vi "运维调试_氨氮.vi"() -> ()   [LabVIEW 2016, in "氨氮.lvlib"]
uses:
  <vilib>/Platform/TimedLoop/XDataNode/timing_clust.ctl
  <vilib>/Platform/TimedLoop/XDataNode/nitl_modes.ctl
  <vilib>/Platform/TimedLoop/XDataNode/wakeup.ctl
  <vilib>/Utility/miscctls.llb/LVPointTypeDef.ctl
  <vilib>/Platform/TimedLoop/XDataNode/XDataNode.xnode
  <vilib>/Platform/TimedLoop/XDataNode/XDNodeRunTimeDep.lvlib
panel:
  in  "设置":bool
  in  "返回 2":bool
  out "固件版本号":string
  in  "数组":string[](array[string])
  in  "备用系数写入":bool
  in  "备用系数读取":bool
  in  "备用系数":T1
  in  "量程切换阈值写入":bool
  in  "量程切换阈值读取":bool
  in  "量程切换阈值":cluster{"阈值":dbl, "标液浓度":dbl}
  in  "参数下拉列表":enum16{"氨氮", "总磷"}(ring)
  in  "量程下拉列表":enum16{"低量程", "高量程"}(ring)
  in  "测量模式下拉列表":enum16{"水样测量", "空白核查", "标样核查", "盲样测试", "加标回收"}(ring)
  in  "公式":cluster{"X^2":dbl, "X":dbl, "b":dbl}
  in  "写公式":bool
  in  "读公式":bool
  in  "精度":dbl=4.0
  in  "样品5 F0":dbl
  in  "样品5 F1":dbl
  in  "样品4 F1":dbl
  in  "样品4 F0":dbl
  in  "样品3 F0":dbl
  in  "样品3 F1":dbl
  in  "样品2 F0":dbl
  in  "样品2 F1":dbl
  in  "样品1 F1":dbl
  in  "样品1 F0":dbl
  in  "method":u16(ring) items=["最小二乘", "最小绝对残差", "Bisquare"]
  in  "模型":enum32{"线性", "多项式"}(ring)
  out "r^2":dbl format="%.7g"
  out "拟合公式":string
  in  "样品2启用":bool
  in  "样品5启用":bool
  in  "样品4启用":bool
  in  "样品3启用":bool
  in  "样品1启用":bool
  in  "标液浓度5":dbl
  out "测量吸光度5":dbl
  in  "标液浓度4":dbl
  out "测量吸光度4":dbl
  in  "标液浓度3":dbl
  out "测量吸光度3":dbl
  in  "标液浓度2":dbl
  out "测量吸光度2":dbl
  out "测量吸光度1":dbl
  in  "标液浓度1":dbl
  out "XY图":cluster{"X Values":dbl[], "Y Values":dbl[]}[](graph)
  in  "返回":bool
  in  "调试":bool
  out "序列号":string="序列号"
  out "氨氮测量数据":T2(xcontrol)
  out "集成报警信息":string
  out "设置值":dbl
  out "定时启动":bool
  out "总磷总氮运行状态":T3(xcontrol)
  in  "停止":bool
  in  "手动启动":bool
  in  "单步测试":bool
  in  "总磷氨氮调试":u16[](xcontrol)
  out "F3":sgl format="%#.6f"
  out "F2":sgl format="%#.6f"
  out "F1":sgl format="%#.6f"
  out "F0":sgl format="%#.6f"
  out "多列列表框":i32(listbox)
  # "COM1"
  # "参数设置"
  # "标液浓度"
  # "F0"
  # "F1"
  # "吸光值显示"
  # "辅\n助\n计\n算\n区"
  # "样品一"
  # "样品二"
  # "样品三"
  # "样品四"
  # "样品五"
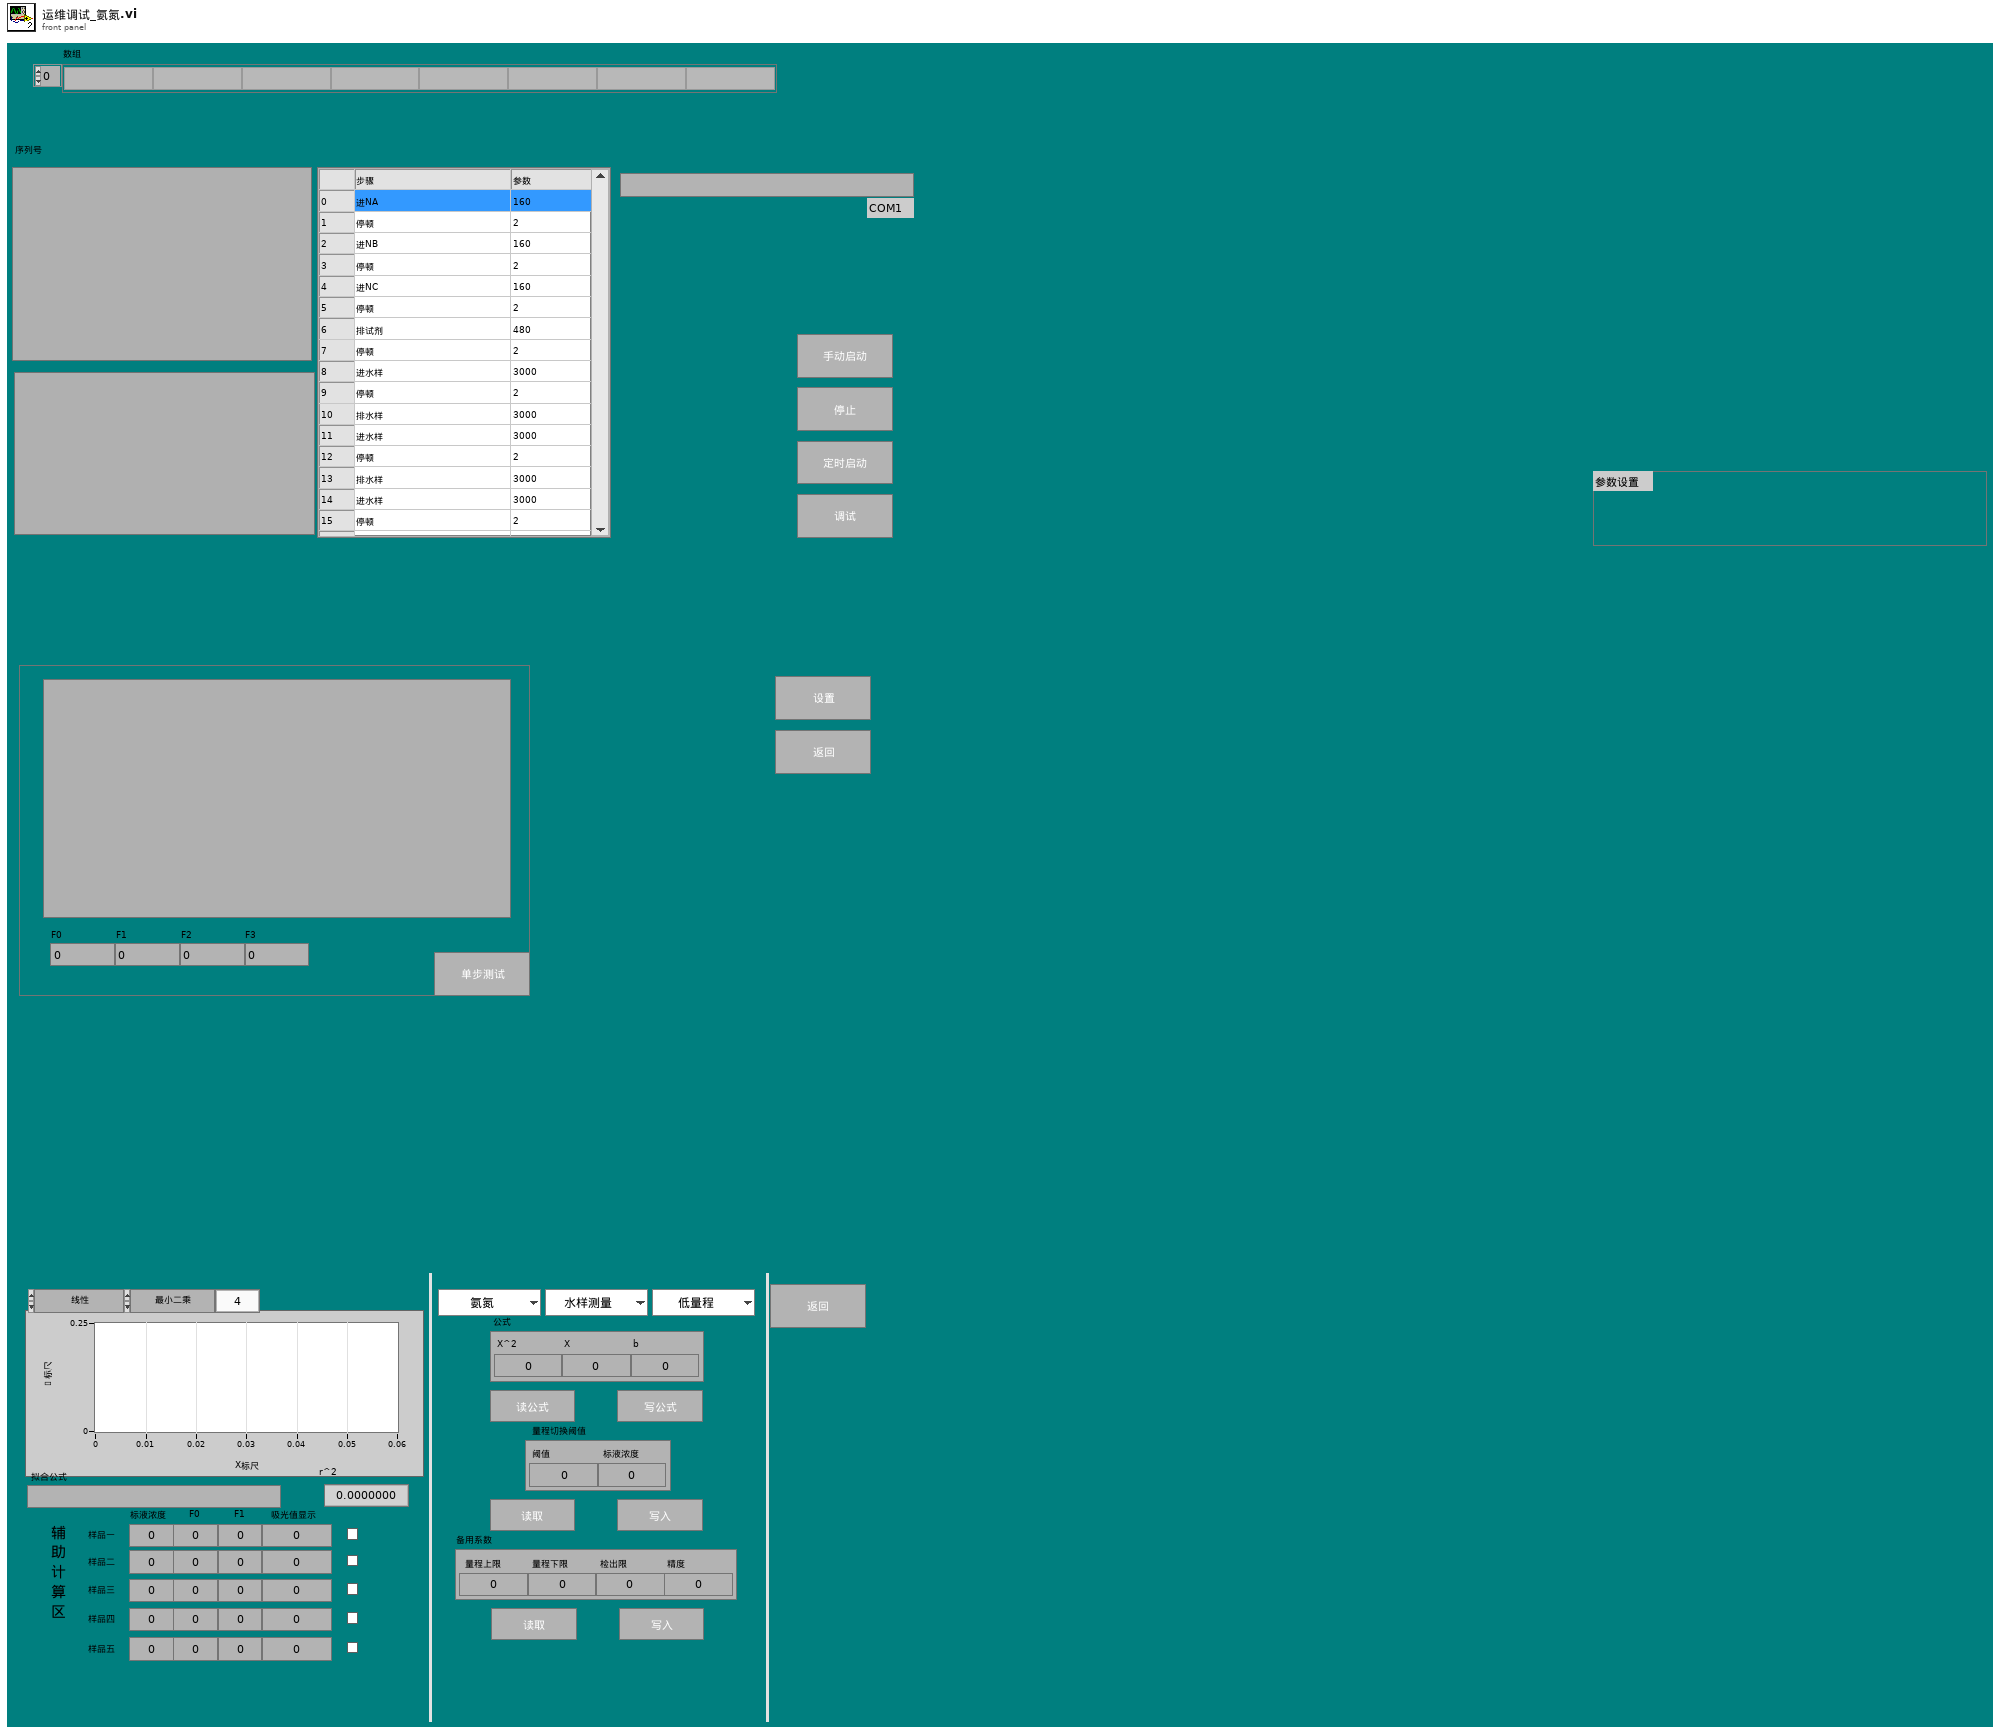
[diagram p1: front panel]
types:
  T1 = cluster{"量程上限":dbl, "量程下限":dbl, "检出限":dbl, "精度":dbl}
  T2 = cluster{"flowid":u16, "测量精度":u16, "测量数据区":cluster{"因子编码":u32, "单位":u16, "标样参考值":sgl, "水样数据时间":timestamp, "水样实测值":sgl, "水样数据标识":string, "标样数据时间":timestamp, "标样实测值":sgl, "标样数据标识":string, "空白数据时间":timestamp, "空白实测值":sgl, "空白数据标识":string, "零点核查数据时间":timestamp, "零点核查实测值":sgl, "零点核查数据标识":string, "跨度核查数据时间":timestamp, "跨度核查实测值":sgl, "跨度核查数据标识":string, "加标回收数据时间":timestamp, "加标回收实测值":sgl, "加标回收数据标识":string, "平行样数据时间":timestamp, "平行样实测值":sgl, "平行样数据标识":string}}
  T3 = cluster{"系统时间":timestamp, "工作状态":enum16{"空闲", "水样测试", "标样核查", "零点核查", "跨度核查", "空白测试", "平行样测试", "加标回收", "空白校准", "标样校准", "初始化（清洗）"}, "测量模式":enum16{"待机", "连续模式", "周期模式", "定点模式", "受控模式", "手动模式"}, "告警代码":enum16{"无告警", "缺试剂告警", "缺水样告警", "缺蒸馏水告警", "缺标液告警", "仪表漏液告警", "标定异常告警", "超量程告警", "加热异常", "低试剂预警", "超上限告警", "超下限告警", "仪表内部其他异常", "滴定异常告警", "电极异常告警", "量程切换告警", "参数设置告警", "PH电极电位异常", "电导率电极异常", "浊度光度异常", "溶解氧电极异常", "溶解氧光强异常", "温度异常告警", "PH异常告警", "溶解氧异常告警", "电导率异常告警", "浊度异常告警", "叶绿素异常告警", "藻密度异常告警", "蓝绿藻异常告警", "ORP异常告警", "氨氮异常告警", "清洁刷异常告警", "SD卡异常告警", "蓝牙异常告警", "Wifi异常告警", "流程异常告警"}, "故障代码":enum16{"无故障", "电机故障", "温度故障", "通讯故障", "滴定故障"}, "日志代码":u16, "软件版本":u16, "F0":sgl, "F1":sgl, "F2":sgl, "F3":sgl, "T":sgl, "H":sgl, "id":u16, "flowid":u16, "量程":u16}
  T4 = enum16{"待机", "启动氨氮", "氨氮测量中", "启动总磷", "总磷测量中", "延时"}
  T5 = typedef "LVPointTypeDef.ctl" = cluster{"Horizontal":i16, "Vertical":i16}
  T6 = cluster{"因子编码":u32, "单位":u16, "标样参考值":sgl, "水样数据时间":timestamp, "水样实测值":sgl, "水样数据标识":string, "标样数据时间":timestamp, "标样实测值":sgl, "标样数据标识":string, "空白数据时间":timestamp, "空白实测值":sgl, "空白数据标识":string, "零点核查数据时间":timestamp, "零点核查实测值":sgl, "零点核查数据标识":string, "跨度核查数据时间":timestamp, "跨度核查实测值":sgl, "跨度核查数据标识":string, "加标回收数据时间":timestamp, "加标回收实测值":sgl, "加标回收数据标识":string, "平行样数据时间":timestamp, "平行样实测值":sgl, "平行样数据标识":string}
  T7 = enum16{"空闲", "水样测试", "标样核查", "零点核查", "跨度核查", "空白测试", "平行样测试", "加标回收", "空白校准", "标样校准", "初始化（清洗）"}
  T8 = cluster{"启动模式":enum16{"标液测量", "水样测量", "零液测量", "盲样测量", "加标回收"}, "启动参数":u16, "量程":enum16{"低量程", "高量程"}}
  T9 = cluster{"时间标识":timestamp, "设备":string, "日志信息":string, "流程参数":string}
  T10 = cluster{"时间标识":timestamp, "设备":string, "日志信息":string}
  T11 = enum16{"无告警", "缺试剂告警", "缺水样告警", "缺蒸馏水告警", "缺标液告警", "仪表漏液告警", "标定异常告警", "超量程告警", "加热异常", "低试剂预警", "超上限告警", "超下限告警", "仪表内部其他异常", "滴定异常告警", "电极异常告警", "量程切换告警", "参数设置告警", "PH电极电位异常", "电导率电极异常", "浊度光度异常", "溶解氧电极异常", "溶解氧光强异常", "温度异常告警", "PH异常告警", "溶解氧异常告警", "电导率异常告警", "浊度异常告警", "叶绿素异常告警", "藻密度异常告警", "蓝绿藻异常告警", "ORP异常告警", "氨氮异常告警", "清洁刷异常告警", "SD卡异常告警", "蓝牙异常告警", "Wifi异常告警", "流程异常告警"}
  T12 = typedef "LVRowAndColumnUnsignedTypeDef.ctl" = cluster{"Row":u32, "Column":u32}
  T13 = typedef "XDNodeRunTimeDep.lvlib/timing_clust.ctl" = cluster{"Expected End [f-1]":u64, "Actual End [f-1]":u64, "Finished Late? [f-1]":bool, "Expected End [i-1]":u64, "Actual End [i-1]":u64, "Finished Late? [i-1]":bool, "Expected Start [i]":u64, "Actual Start [i]":u64, "Expected Start [f]":u64, "Actual Start [f]":u64, "Source Name":string, "Structure Name":string, "Period":i64, "Deadline":i64, "Offset":i64, "Start":i64, "Priority":i32, "Timeout":i32, "Mode":T14, "Wakeup Reason":T15, "Error":errorcluster, "Source Type":string, "Secondary Source Type":string, "Global End Time":u64, "Global Start Time":u64, "Frame Duration":u64, "Iteration Duration":u64, "Assigned CPU":i32, "I/O Scan Engine Mode":u32}
  T14 = typedef "XDNodeRunTimeDep.lvlib/nitl_modes.ctl" = enum32{"No Change", "Process missed periods, maintain original phase", "Discard missed periods, maintain original phase", "Process missed periods, ignore original phase", "Discard missed periods, ignore original phase"}
  T15 = typedef "XDNodeRunTimeDep.lvlib/wakeup.ctl" = enum32{"Normal", "Aborted", "Asynchronous wakeup", "Timing source error", "Timed loop error", "Timeout"}
  T16 = cluster{"站号":u16, "量程切换":enum32{"H", "L", "AUTO"}, "控制命令":enum16{"启动测量", "标样核查", "零点核查", "跨度核查", "空白测试", "平行样测试", "加标回收", "空白校准", "标样校准", "初始化（清洗）", "停止测试", "仪器重启", "校时", "模式设置", "测量间隔设置", "盲样测试"}, "模式设置":enum16{"待机", "连续模式", "周期模式", "定点模式", "受控模式", "手动模式"}, "测量间隔":u16}
  T17 = cluster{"站号":u16, "量程切换":enum32{"H", "L", "AUTO"}, "控制命令":enum16{"启动测量", "标样核查", "零点核查", "跨度核查", "空白测试", "平行样测试", "加标回收", "空白校准", "标样校准", "初始化（清洗）", "停止测试", "仪器重启", "校时", "模式设置", "测量间隔设置"}, "模式设置":enum16{"待机", "连续模式", "周期模式", "定点模式", "受控模式", "手动模式"}, "测量间隔":u16}
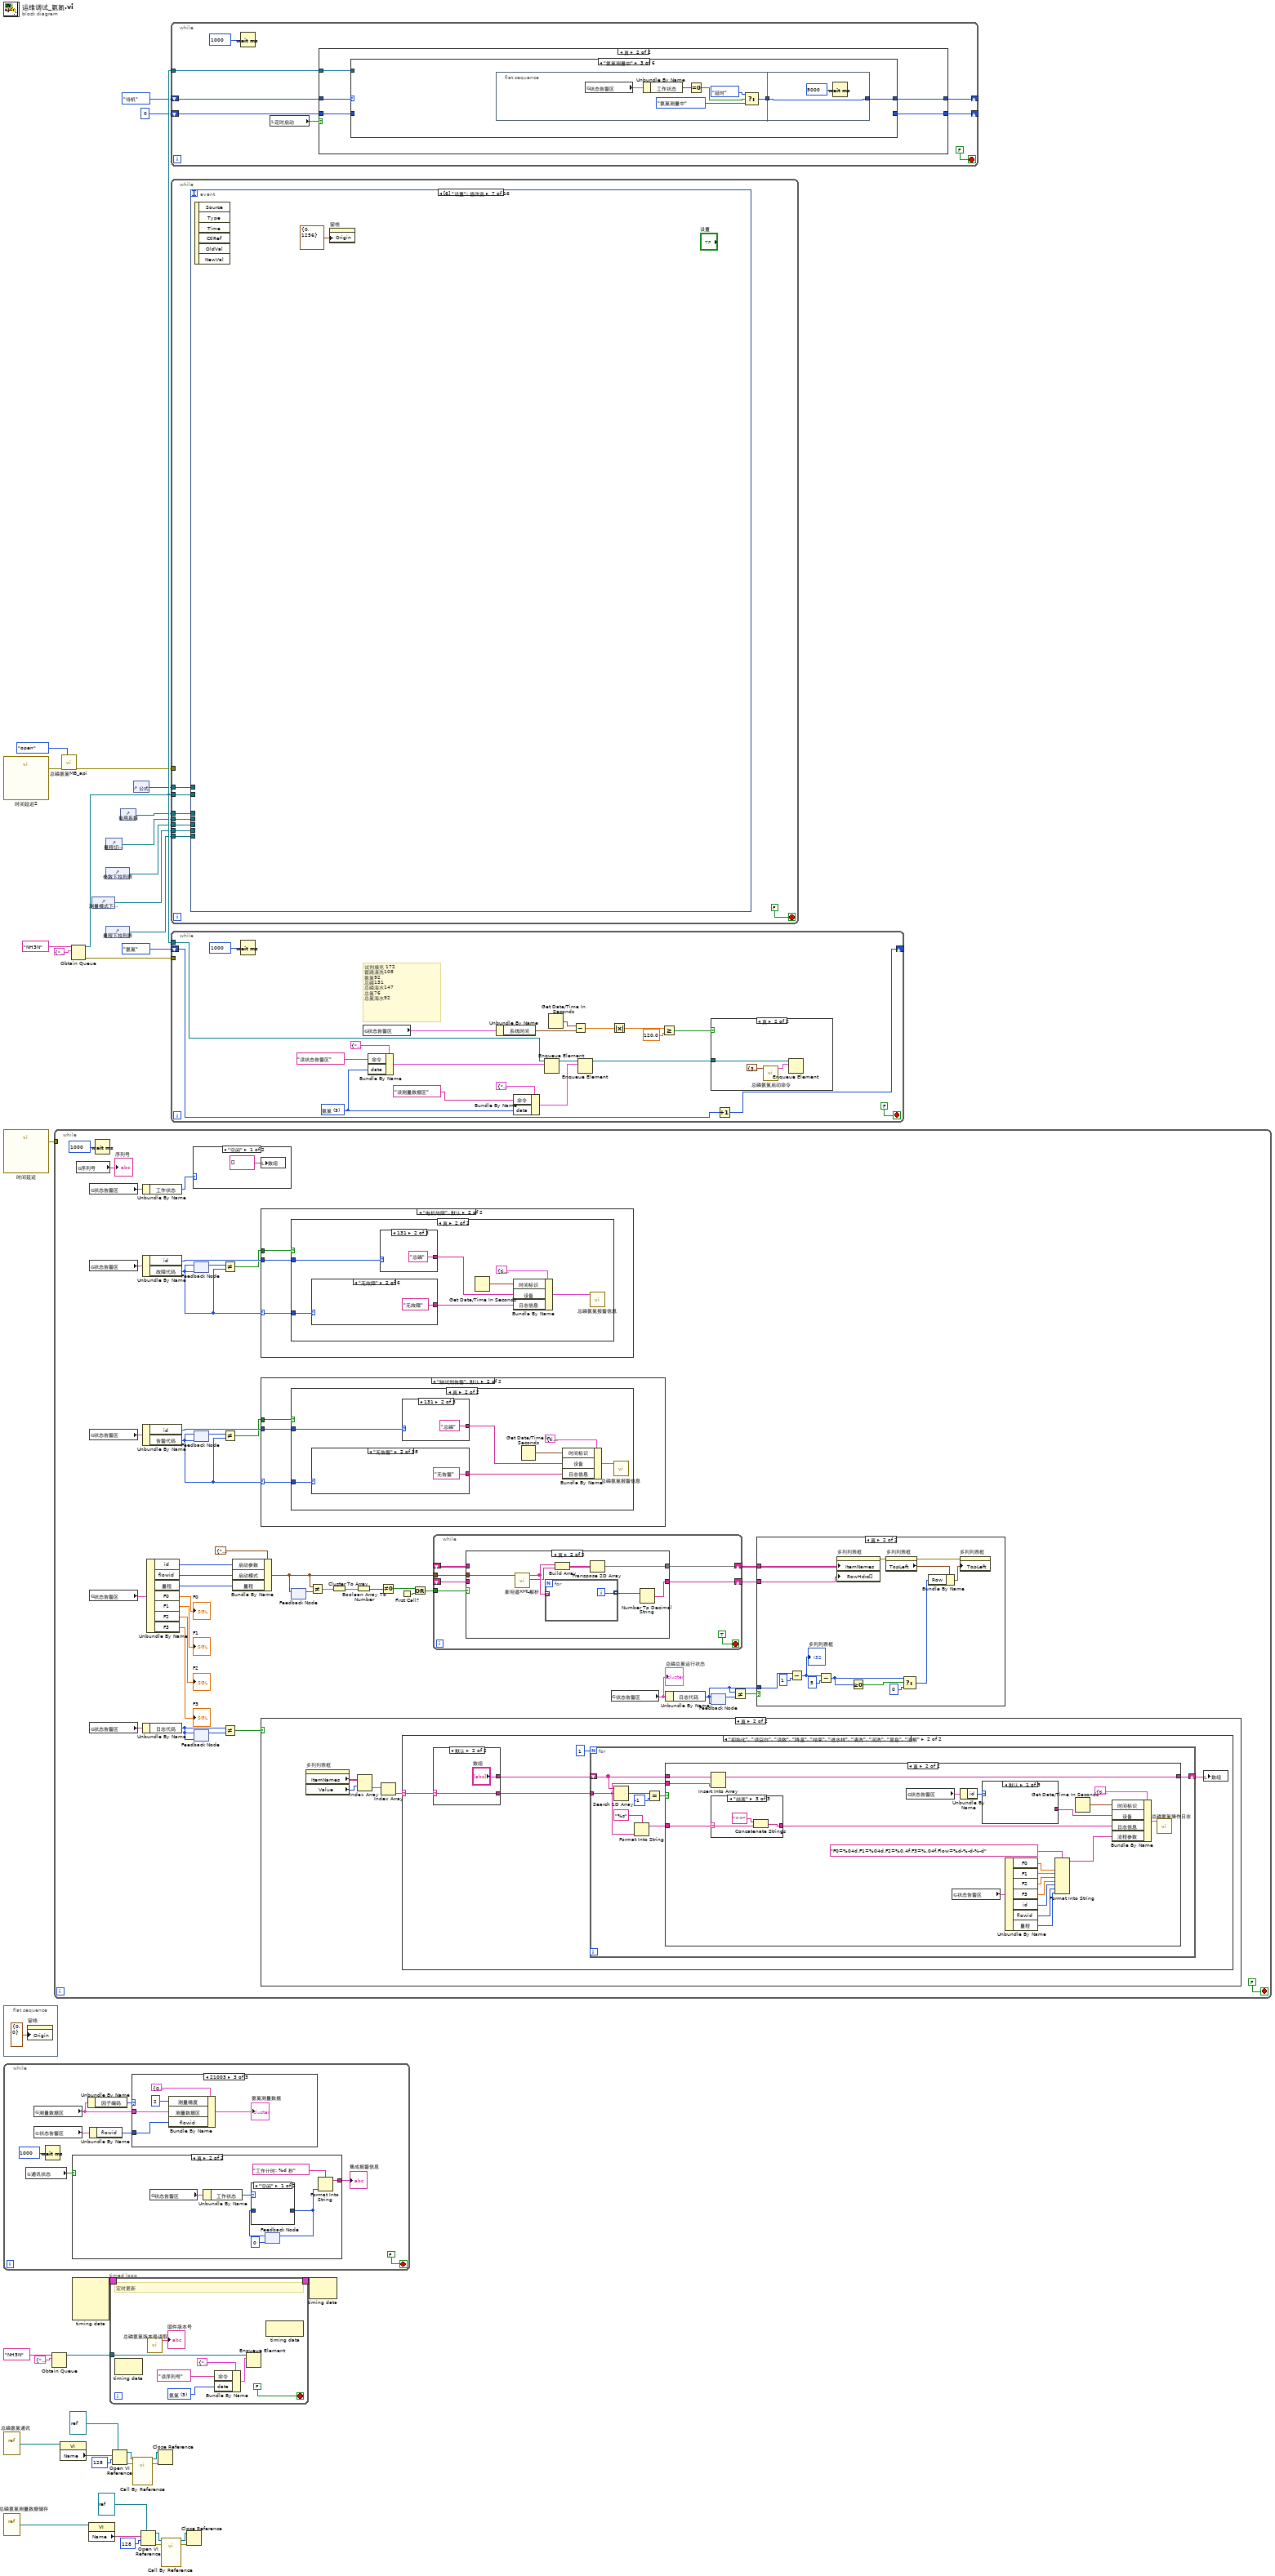
[diagram p0: block diagram]
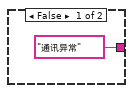
[diagram p2: hidden frame]
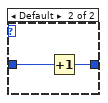
[diagram p3: hidden frame]
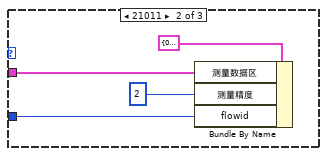
[diagram p5: hidden frame]
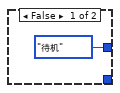
[diagram p6: hidden frame]
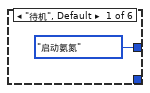
[diagram p7: hidden frame]
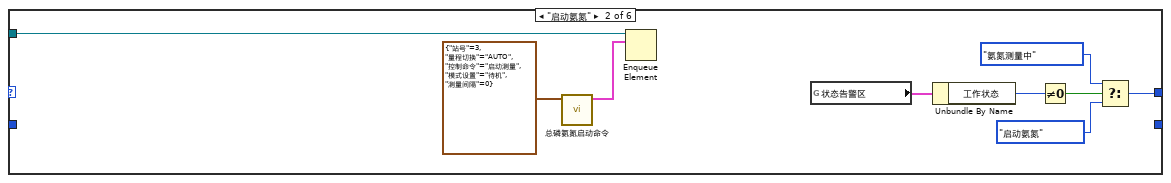
[diagram p8: hidden frame]
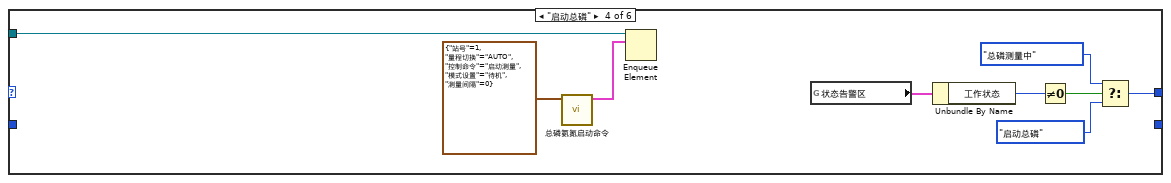
[diagram p9: hidden frame]
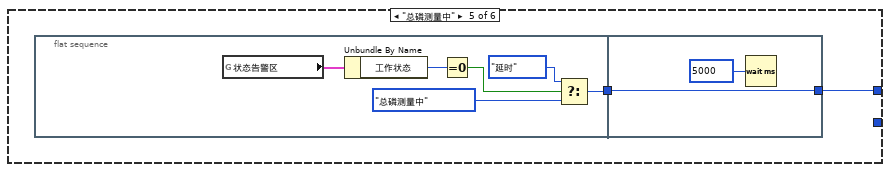
[diagram p10: hidden frame]
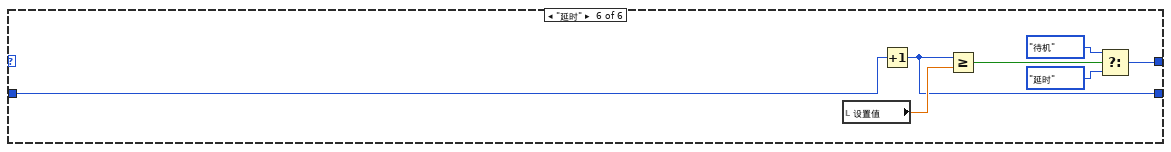
[diagram p11: hidden frame]
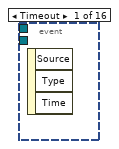
[diagram p12: hidden frame]
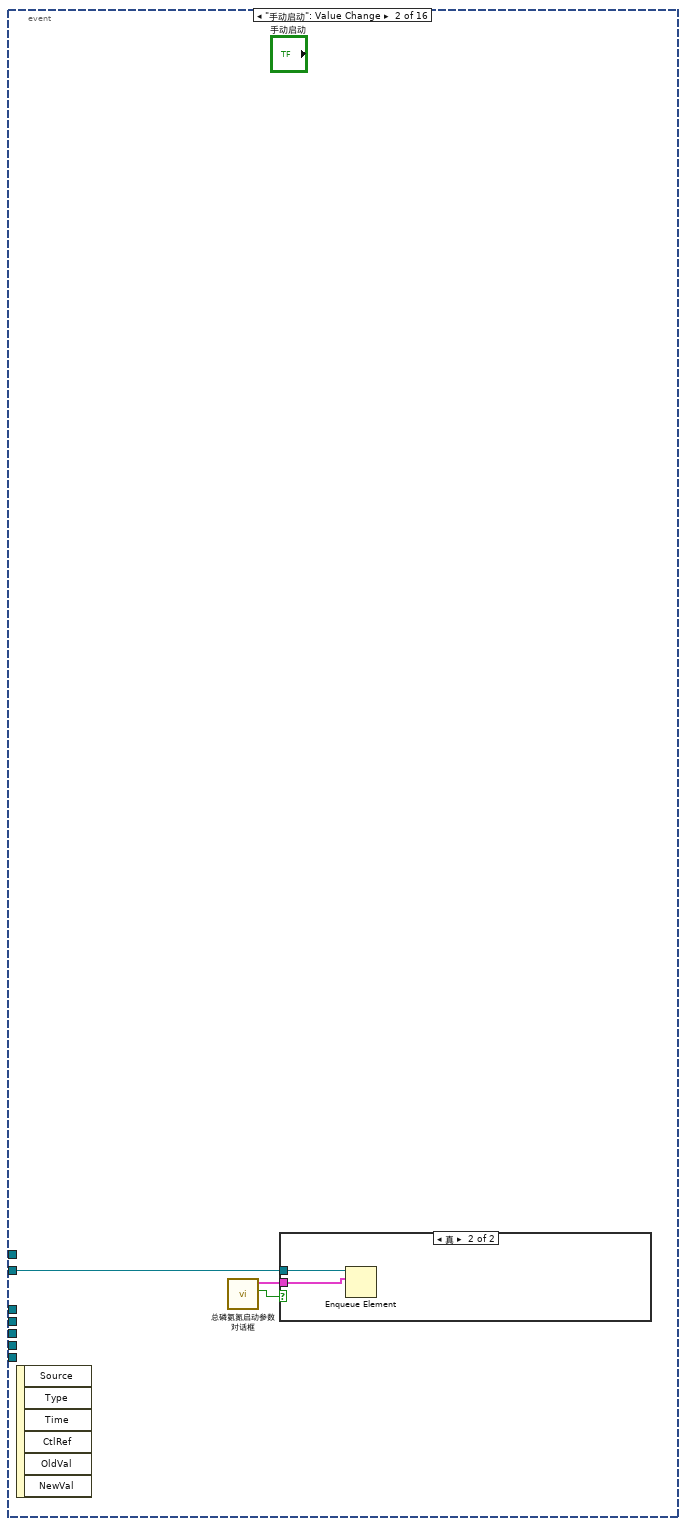
[diagram p13: hidden frame]
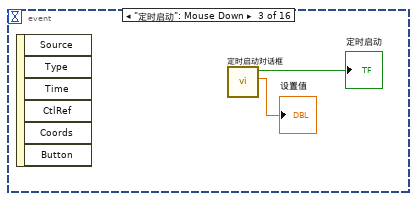
[diagram p15: hidden frame]
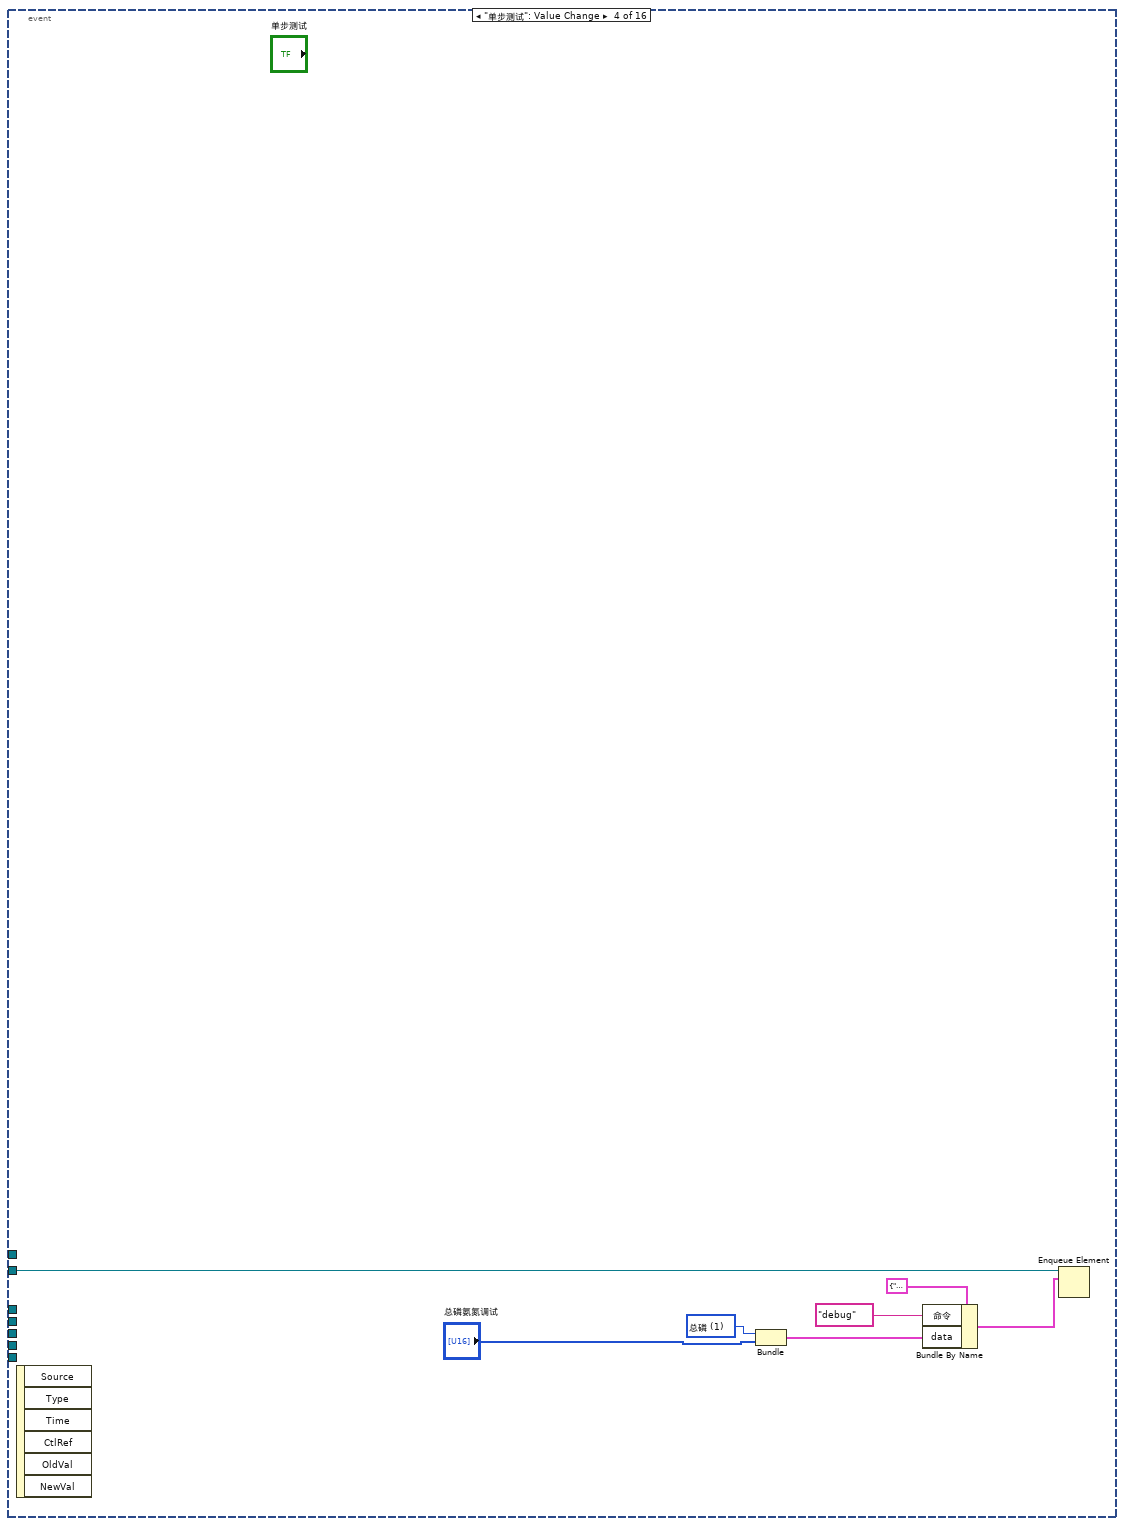
[diagram p16: hidden frame]
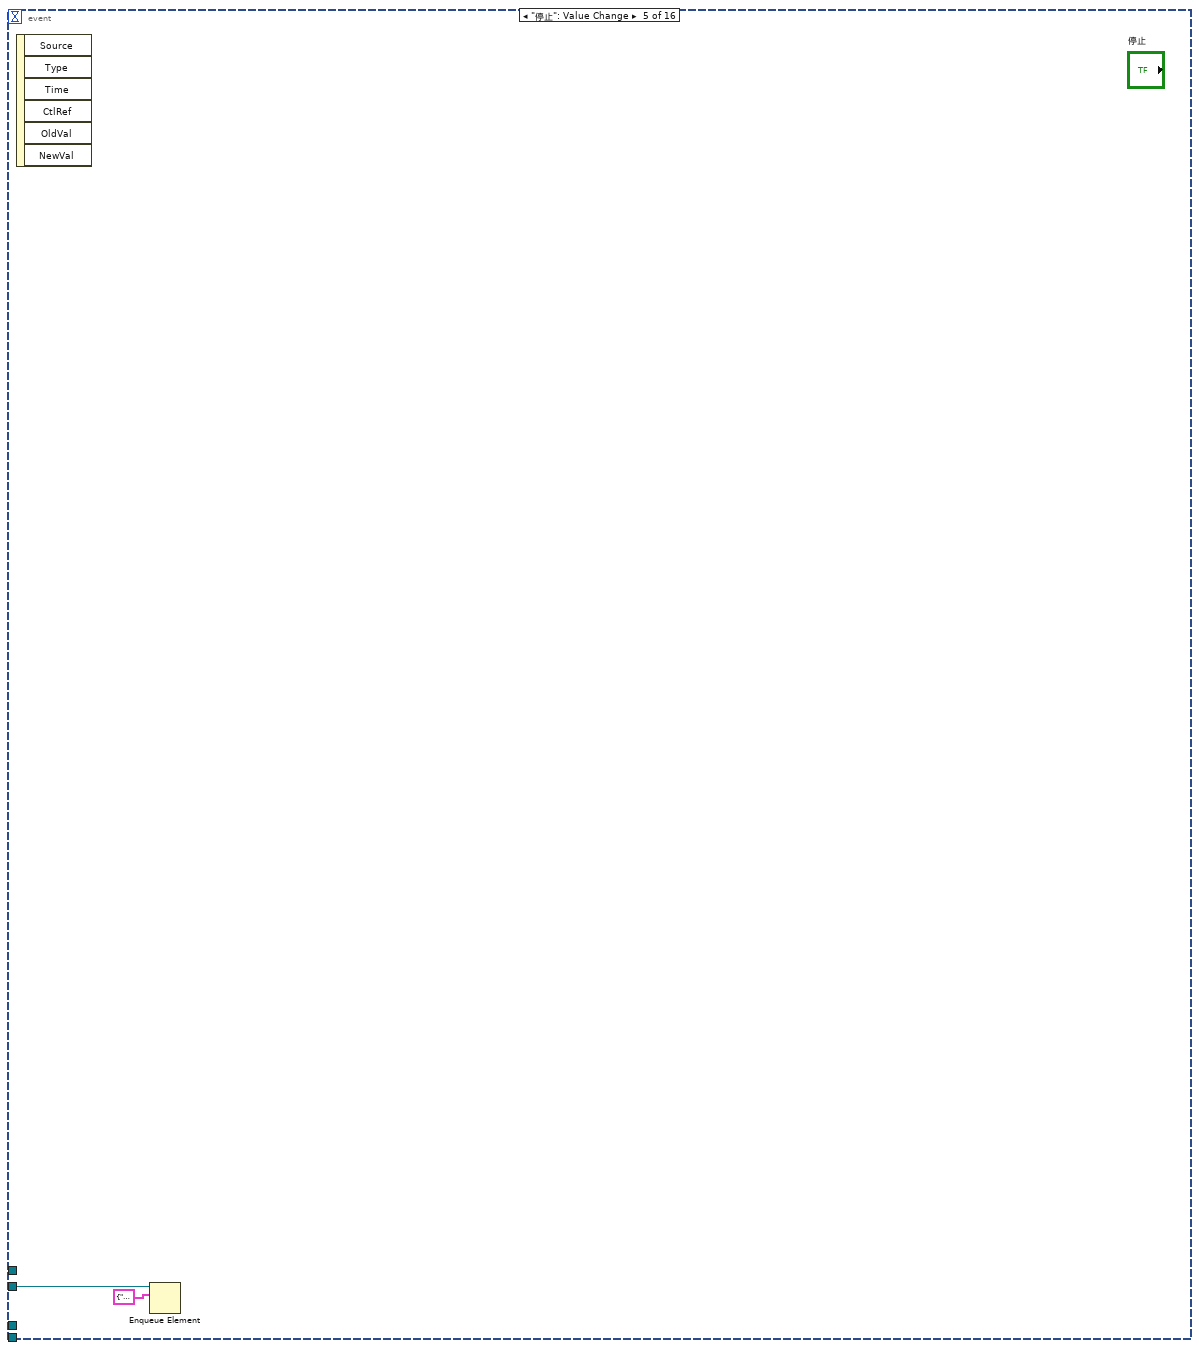
[diagram p17: hidden frame]
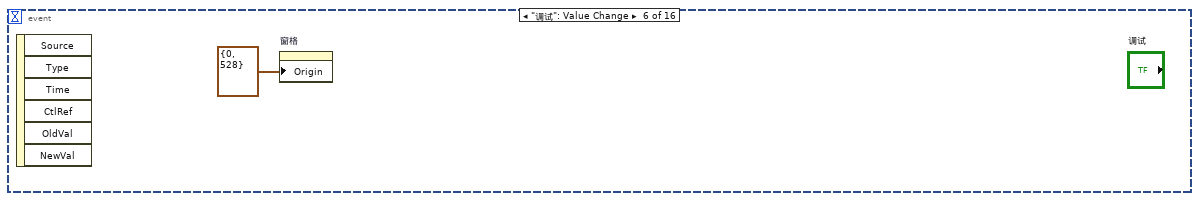
[diagram p18: hidden frame]
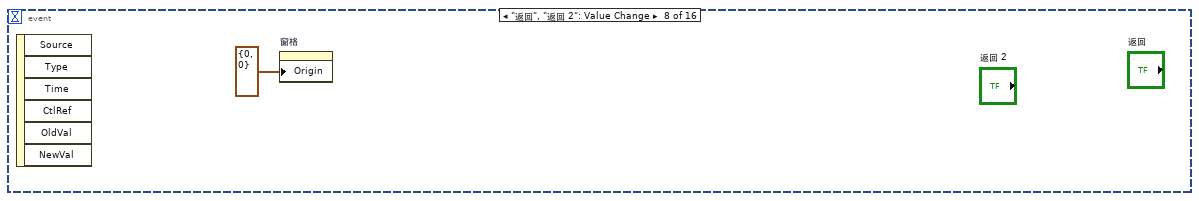
[diagram p19: hidden frame]
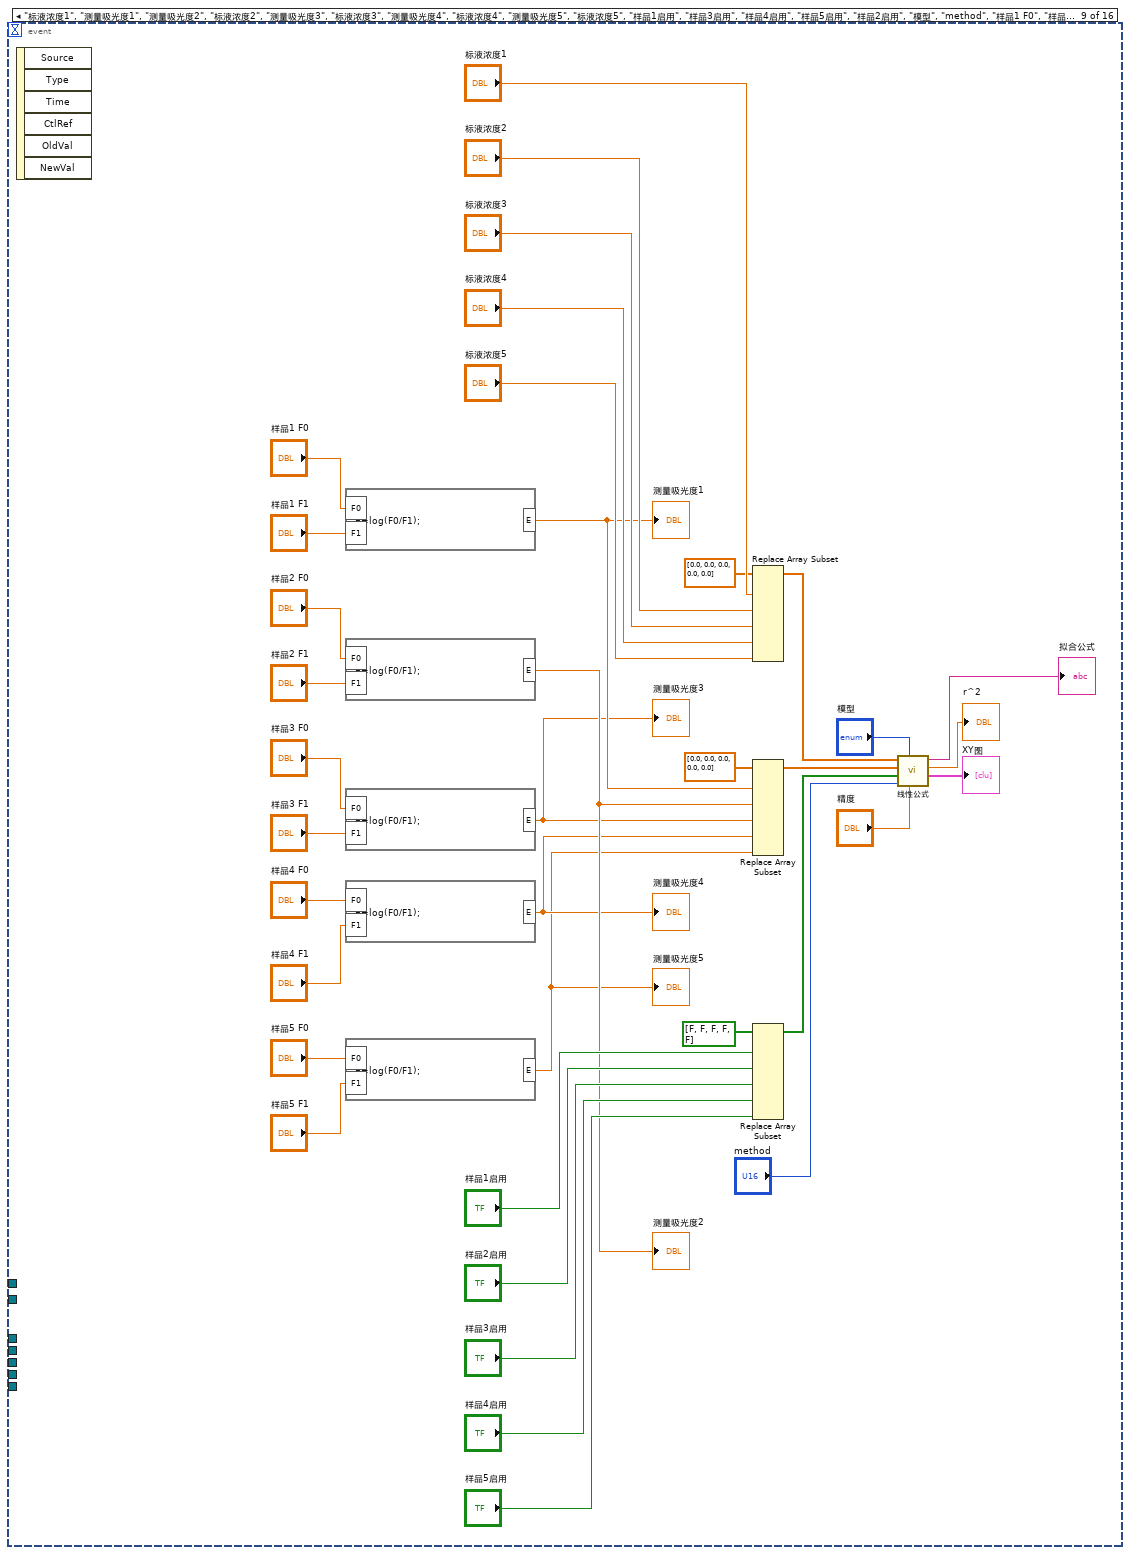
[diagram p20: hidden frame]
diagram:
  n1 = call "时间延迟2"() -> ("error out"=w1:errorcluster)  [unwired: 11 in]
  n2 = call "时间延迟"() -> ("error out"=w9:errorcluster)  [unwired: 11 in]
  n3 = flat-sequence {
    frame #0 {
      n4 = property on="窗格" class="Pane"("Origin"=T5 {"Horizontal"=0, "Vertical"=0} ("原点")) -> ()  [unwired: 2 in, 2 out]
    }
  }
  n5 = while {
    stop <- FALSE stop-if-true
    n6 = global read "VAR总磷氨氮全局变量.vi" "通讯状态"() -> (w43:bool)
    n7 = global read "VAR总磷氨氮全局变量.vi" "测量数据区"() -> (w45:T6)
    n8 = global read "VAR总磷氨氮全局变量.vi" "状态告警区"() -> (w41:T3)
    n9 = Wait (ms)(milliseconds to wait=u32 1000 ("等待时间（毫秒）")) -> ()  [unwired: 1 out]
    n10 = case shown="真" w43 {
      tunnel: ["通讯异常" ("集成报警信息") w49] -> w42
      frame False {
      }
      frame True {
        n11 = global read "VAR总磷氨氮全局变量.vi" "状态告警区"() -> (w55:T3)
        n12 = Unbundle By Name(w55) -> ("工作状态"=w54:T7)
        n13 = feedback #1(0) -> (w52:i32)
        n14 = case shown="\"空闲\"" w54 {
          tunnel: w52 -> [_ w57]
          tunnel: [_ w56] -> w50
          frame "空闲" {
          }
          frame Default {
            n15 = Increment(x=w57) -> (x+1=w56:i32)
          }
        }
        n16 = feedback-in #1(w50) -> ()
        n17 = Format Into String(format string="工作计时: %d 秒" ("格式字符串"), w50) -> (resulting string=w49:string)  [unwired: 2 in, 1 out]
      }
    }
    "集成报警信息" <- w42
    n18 = Unbundle By Name(w45) -> ("因子编码"=w44:u32)
    n19 = Unbundle By Name(w41) -> ("flowid"=w40:u16)
    n20 = case shown="21003" w44 {
      tunnel: w45 -> [_ w61 w66]
      tunnel: w40 -> [_ w59 w64]
      frame Default {
      }
      frame 21011 {
        n21 = Bundle By Name(cluster=T2 {"flowid"=0, "测量精度"=0, "测量数据区"={"因子编码"=0, "单位"=0, "标样参考值"=0.0, "水样数据时间"=timestamp(0 s since 1904-01-01), "水样实测值"=0.0, "水样数据标识"="", "标样数据时间"=timestamp(0 s since 1904-01-01), "标样实测值"=0.0, "标样数据标识"="", "空白数据时间"=timestamp(0 s since 1904-01-01), "空白实测值"=0.0, "空白数据标识"="", "零点核查数据时间"=timestamp(0 s since 1904-01-01), "零点核查实测值"=0.0, "零点核查数据标识"="", "跨度核查数据时间"=timestamp(0 s since 1904-01-01), "跨度核查实测值"=0.0, "跨度核查数据标识"="", "加标回收数据时间"=timestamp(0 s since 1904-01-01), "加标回收实测值"=0.0, "加标回收数据标识"="", "平行样数据时间"=timestamp(0 s since 1904-01-01), "平行样实测值"=0.0, "平行样数据标识"=""}} ("氨氮测量数据"), "测量数据区"=w61, "测量精度"=u16 2, "flowid"=w59) -> ()  [unwired: 1 out]
      }
      frame 21003 {
        n22 = Bundle By Name(cluster=T2 {"flowid"=0, "测量精度"=0, "测量数据区"={"因子编码"=0, "单位"=0, "标样参考值"=0.0, "水样数据时间"=timestamp(0 s since 1904-01-01), "水样实测值"=0.0, "水样数据标识"="", "标样数据时间"=timestamp(0 s since 1904-01-01), "标样实测值"=0.0, "标样数据标识"="", "空白数据时间"=timestamp(0 s since 1904-01-01), "空白实测值"=0.0, "空白数据标识"="", "零点核查数据时间"=timestamp(0 s since 1904-01-01), "零点核查实测值"=0.0, "零点核查数据标识"="", "跨度核查数据时间"=timestamp(0 s since 1904-01-01), "跨度核查实测值"=0.0, "跨度核查数据标识"="", "加标回收数据时间"=timestamp(0 s since 1904-01-01), "加标回收实测值"=0.0, "加标回收数据标识"="", "平行样数据时间"=timestamp(0 s since 1904-01-01), "平行样实测值"=0.0, "平行样数据标识"=""}} ("氨氮测量数据"), "测量精度"=u16 2, "测量数据区"=w66, "flowid"=w64) -> (→"氨氮测量数据":T2)
      }
    }
  }
  n23 = vi-ref "总磷氨氮通讯.vi"() -> (w32:refnum<vi>)
  n24 = vi-ref "总磷氨氮测量数据储存.vi"() -> (w24:refnum<vi>)
  n25 = Obtain Queue(name (unnamed)="NH3N" ("名称（未命名）"), element data type=cluster{"命令":string, "data":variant} {"命令"="", "data"=variant}) -> (queue out=w2:refnum<queue>)  [unwired: 3 in, 2 out]
  n26 = while {
    tunnel: w9 -> [_]
    stop <- FALSE stop-if-true
    n27 = global read "VAR总磷氨氮全局变量.vi" "序列号"() -> (→"序列号":string)
    n28 = global read "VAR总磷氨氮全局变量.vi" "状态告警区"() -> (w72:T3)
    n29 = global read "VAR总磷氨氮全局变量.vi" "状态告警区"() -> (w78:T3)
    n30 = global read "VAR总磷氨氮全局变量.vi" "状态告警区"() -> (w83:T3)
    n31 = global read "VAR总磷氨氮全局变量.vi" "状态告警区"() -> (w95:T3)
    n32 = global read "VAR总磷氨氮全局变量.vi" "状态告警区"() -> (w69:T3)
    n33 = Wait (ms)(milliseconds to wait=u32 1000 ("等待时间（毫秒）")) -> ()  [unwired: 1 out]
    n34 = Unbundle By Name(w72) -> ("工作状态"=w71:T7)
    n35 = Unbundle By Name(w78) -> ("id"=w77:u16, "故障代码"=w74:enum16{"无故障", "电机故障", "温度故障", "通讯故障", "滴定故障"})
    n36 = Unbundle By Name(w83) -> ("id"=w82:u16, "告警代码"=w79:T11)
    n37 = Unbundle By Name(w69) -> ("日志代码"=w68:u16)
    n38 = Unbundle By Name(w95) -> ("id"=w92:u16, "flowid"=w94:u16, "量程"=w93:u16, "F0"=→"F0":sgl, "F1"=→"F1":sgl, "F2"=→"F2":sgl, "F3"=→"F3":sgl)
    n39 = case shown="\"空闲\"" w71 {
      frame "空闲" {
        n40 = local write "数组"(string[] [] ("数组")) -> ()
      }
      frame "水样测试", Default {
      }
    }
    n41 = feedback #2(w74) -> (w75:enum16{"无故障", "电机故障", "温度故障", "通讯故障", "滴定故障"})
    n42 = feedback-in #2(w74) -> ()
    n43 = feedback #3(w79) -> (w80:T11)
    n44 = feedback-in #3(w79) -> ()
    n45 = feedback #4(w68) -> (w70:u16)
    n46 = feedback-in #4(w68) -> ()
    n47 = Not Equal?(x=w75, y=w74) -> (x != y?=w76:bool)
    n48 = Not Equal?(x=w80, y=w79) -> (x != y?=w81:bool)
    n49 = Not Equal?(x=w68, y=w70) -> (x != y?=w67:bool)
    n50 = Bundle By Name(cluster=T8 {"启动模式"=enum."加标回收", "启动参数"=1, "量程"=enum."低量程"} ("参数簇"), "启动参数"=w92, "启动模式"=w94, "量程"=w93) -> (w85:T8)
    n51 = case shown="\"电机故障\", 默认" w74 {
      selector: w74 -> [_ w163]
      tunnel: w77 -> [_ w164]
      tunnel: w76 -> [_ w162]
      frame "无故障" {
      }
      frame "电机故障", Default {
        n52 = case shown="真" w162 {
          tunnel: w164 -> [_ w171]
          tunnel: w163 -> [_ w166]
          frame False {
          }
          frame True {
            n53 = case shown="\"无故障\"" w166 {
              selector: w166 -> [w173 _ _ _ _ _]
              tunnel: [w172 "无故障" "电机故障" "温度故障" "通讯故障" "滴定故障"] -> w165
              frame Default {
                n54 = Format Into String(format string="%d" ("格式字符串"), initial string="未知" ("工作状态"), w173) -> (resulting string=w172:string)  [unwired: 1 in, 1 out]
              }
              frame "无故障" {
              }
              frame "电机故障" {
              }
              frame "温度故障" {
              }
              frame "通讯故障" {
              }
              frame "滴定故障" {
              }
            }
            n55 = case shown="131" w171 {
              tunnel: [_ "总磷" ("table输入") "氨氮" ("table输入")] -> w167
              frame Default {
              }
              frame 131 {
              }
              frame 92 {
              }
            }
            n56 = Get Date/Time In Seconds() -> (seconds since 1Jan1904=w168:timestamp)
            n57 = Bundle By Name(cluster=T10 {"时间标识"=timestamp(0 s since 1904-01-01), "设备"="", "日志信息"=""} ("data in"), "时间标识"=w168, "设备"=w167, "日志信息"=w165) -> (w169:T10)
            n58 = call "总磷氨氮报警信息.vi"("data in"=w169) -> ()  [unwired: 11 in]
          }
        }
      }
    }
    n59 = case shown="\"缺试剂告警\", 默认" w79 {
      selector: w79 -> [_ w184]
      tunnel: w82 -> [_ w185]
      tunnel: w81 -> [_ w183]
      frame "无告警" {
      }
      frame "缺试剂告警", Default {
        n60 = case shown="真" w183 {
          tunnel: w185 -> [_ w192]
          tunnel: w184 -> [_ w186]
          frame False {
          }
          frame True {
            n61 = case shown="\"无告警\"" w186 {
              selector: w186 -> [w194 _ _ _ _ _ _ _ _ _ _ _ _ _ _ _ _ _ _ _ _ _ _ _ _ _ _ _ _ _ _ _ _ _ _ _ _ _]
              tunnel: [w193 "无告警" "缺试剂告警" "缺水样告警" "缺蒸馏水告警" "缺标液告警" "仪表漏液告警" "标定异常告警" "超量程告警" "加热异常" "低试剂预警" "超上限告警" "超下限告警" "仪表内部其他异常" "滴定异常告警" "电极异常告警" "量程切换告警" "参数设置告警" "PH电极电位异常" "电导率电极异常" "浊度光度异常" "溶解氧电极异常" "溶解氧光强异常" "温度异常告警" "PH异常告警" "溶解氧异常告警" "电导率异常告警" "浊度异常告警" "叶绿素异常告警" "藻密度异常告警" "蓝绿藻异常告警" "ORP异常告警" "氨氮异常告警" "清洁刷异常告警" "SD卡异常告警" "蓝牙异常告警" "WiFi异常告警" "流程异常告警"] -> w187
              frame Default {
                n62 = Format Into String(format string="%d" ("格式字符串"), initial string="未知" ("工作状态"), w194) -> (resulting string=w193:string)  [unwired: 1 in, 1 out]
              }
              frame "无告警" {
              }
              frame "缺试剂告警" {
              }
              frame "缺水样告警" {
              }
              frame "缺蒸馏水告警" {
              }
              frame "缺标液告警" {
              }
              frame "仪表漏液告警" {
              }
              frame "标定异常告警" {
              }
              frame "超量程告警" {
              }
              frame "加热异常" {
              }
              frame "低试剂预警" {
              }
              frame "超上限告警" {
              }
              frame "超下限告警" {
              }
              frame "仪表内部其他异常" {
              }
              frame "滴定异常告警" {
              }
              frame "电极异常告警" {
              }
              frame "量程切换告警" {
              }
              frame "参数设置告警" {
              }
              frame "PH电极电位异常" {
              }
              frame "电导率电极异常" {
              }
              frame "浊度光度异常" {
              }
              frame "溶解氧电极异常" {
              }
              frame "溶解氧光强异常" {
              }
              frame "温度异常告警" {
              }
              frame "PH异常告警" {
              }
              frame "溶解氧异常告警" {
              }
              frame "电导率异常告警" {
              }
              frame "浊度异常告警" {
              }
              frame "叶绿素异常告警" {
              }
              frame "藻密度异常告警" {
              }
              frame "蓝绿藻异常告警" {
              }
              frame "ORP异常告警" {
              }
              frame "氨氮异常告警" {
              }
              frame "清洁刷异常告警" {
              }
              frame "SD卡异常告警" {
              }
              frame "蓝牙异常告警" {
              }
              frame "Wifi异常告警" {
              }
              frame "流程异常告警" {
              }
            }
            n63 = case shown="131" w192 {
              tunnel: [_ "总磷" ("table输入") "氨氮" ("table输入")] -> w188
              frame Default {
              }
              frame 131 {
              }
              frame 92 {
              }
            }
            n64 = Get Date/Time In Seconds() -> (seconds since 1Jan1904=w189:timestamp)
            n65 = Bundle By Name(cluster=T10 {"时间标识"=timestamp(0 s since 1904-01-01), "设备"="", "日志信息"=""} ("data in"), "时间标识"=w189, "设备"=w188, "日志信息"=w187) -> (w190:T10)
            n66 = call "总磷氨氮报警信息.vi"("data in"=w190) -> ()  [unwired: 11 in]
          }
        }
      }
    }
    n67 = case shown="真" w67 {
      frame False {
      }
      frame True {
        n68 = property on="多列列表框" class="MCListbox (严格)"() -> ("ItemNames"=w112:string[][], "Value"=w113:i32)  [unwired: 2 in, 2 out]
        n69 = Index Array(array=w112, index (row)=w113) -> (element=w111:string[])  [unwired: 1 in]
        n70 = Index Array(array=w111) -> (element=w110:string)  [unwired: 1 in]
        n71 = case shown="\"初始化\", \"读空白\", \"读数\", \"降温\", \"结束\", \"进水样\", \"清洗\", \"润洗\", \"显色\", \"消解\"" w110 {
          selector: w110 -> [_ w116]
          frame Default {
          }
          frame "初始化", "读空白", "读数", "降温", "结束", "进水样", "清洗", "润洗", "显色", "消解" {
            n72 = case shown="默认" w116 {
              selector: w116 -> [w120 w122]
              tunnel: [w120 w122] -> w115
              tunnel: [string[] [] ("数组") "数组"] -> w114
              frame "读数" {
              }
              frame Default {
              }
            }
            n73 = for {
              N: 1 -> [_]
              tunnel: w115 -> [w124]
              shift-right: [w123] -> w117
              shift-left: w114 -> [w125]
              n74 = Search 1D Array(1D array=w125, element=w124) -> (index of element=w128:i32)  [unwired: 1 in]
              n75 = Format Into String(format string="%s" ("格式字符串"), w124) -> (resulting string=w129:string)  [unwired: 2 in, 1 out]
              n76 = Equal?(x=w128, y=-1) -> (x = y?=w126:bool)
              n77 = case shown="真" w126 {
                tunnel: w129 -> [_ w133]
                tunnel: w125 -> [w131 w137]
                tunnel: w124 -> [_ w136]
                tunnel: [w131 w135] -> w123
                frame False {
                }
                frame True {
                  n78 = Insert Into Array(array=w137, new element=w136) -> (w135:string[])  [unwired: 1 in]
                  n79 = case shown="\"结束\"" w133 {
                    selector: w133 -> [w153 w156 w159]
                    tunnel: [w153 w155 w158] -> w132
                    frame Default {
                    }
                    frame "初始化" {
                      n80 = Concatenate Strings("<<" ("字符串"), w156) -> (w155:string)
                    }
                    frame "结束" {
                      n81 = Concatenate Strings(">>" ("字符串"), w159) -> (w158:string)
                    }
                  }
                  n82 = global read "VAR总磷氨氮全局变量.vi" "状态告警区"() -> (w152:T3)
                  n83 = global read "VAR总磷氨氮全局变量.vi" "状态告警区"() -> (w147:T3)
                  n84 = Unbundle By Name(w152) -> ("id"=w151:u16)
                  n85 = case shown="默认" w151 {
                    tunnel: [_ "总磷" ("table输入") "氨氮" ("table输入")] -> w149
                    frame Default {
                    }
                    frame 131 {
                    }
                    frame 92 {
                    }
                  }
                  n86 = Unbundle By Name(w147) -> ("F0"=w144:sgl, "F1"=w143:sgl, "F2"=w142:sgl, "F3"=w141:sgl, "id"=w140:u16, "flowid"=w139:u16, "量程"=w138:u16)
                  n87 = Format Into String(format string="F0=%04d,F1=%04d,F2=%0.4f,F3=%.04f,Flow=%d-%-d-%-d" ("格式字符串"), w144, w143, w142, w141, w140, w139, w138) -> (resulting string=w145:string)  [unwired: 2 in, 1 out]
                  n88 = Get Date/Time In Seconds() -> (seconds since 1Jan1904=w148:timestamp)
                  n89 = Bundle By Name(cluster=T9 {"时间标识"=timestamp(0 s since 1904-01-01), "设备"="", "日志信息"="", "流程参数"=""} ("data in"), "时间标识"=w148, "设备"=w149, "日志信息"=w132, "流程参数"=w145) -> (w150:T9)
                  n90 = call "总磷氨氮操作日志.vi"("data in"=w150) -> ()  [unwired: 11 in]
                }
              }
            }
            n91 = local write "数组"(w117) -> ()
          }
        }
      }
    }
    n92 = feedback #5() -> (w101:T8)  [unwired: 1 in]
    n93 = feedback-in #5(w85) -> ()
    n94 = Not Equal?(x=w85, y=w101) -> (x != y?=w102:cluster{"启动模式":bool, "启动参数":bool, "量程":bool})
    n95 = Cluster To Array(cluster=w102) -> (array=w103:bool[])
    n96 = Boolean Array To Number(Boolean array=w103) -> (number=w104:u32)
    n97 = Not Equal To 0?(x=w104) -> (x != 0?=w97:bool)
    n98 = First Call?() -> (First Call?: T/F=w98:bool)
    n99 = Or(x=w97, y=w98) -> (x .or. y?=w96:bool)
    n100 = while {
      tunnel: w96 -> [w242]
      tunnel: w85 -> [w241]
      shift-right: [w240] -> w100
      shift-left: _ -> [w236]
      shift-right: [w239] -> w99
      shift-left: _ -> [w237]
      stop <- TRUE stop-if-true
      n101 = case shown="真" w242 {
        tunnel: [w244 w251] -> w239
        tunnel: [w243 w250] -> w240
        tunnel: w241 -> [_ w245]
        tunnel: w237 -> [w244 _]
        tunnel: w236 -> [w243 _]
        frame False {
        }
        frame True {
          n102 = call "斯坦道XML解析.vi"("参数簇"=w245) -> ("步骤时间"=w246:string[], "步骤名"=w248:string[])  [unwired: 9 in]
          n103 = for {
            tunnel: w248 -> [_] mode=indexing
            tunnel: [w252] -> w249 mode=indexing
            i -> [w252]
          }
          n104 = Build Array(w248, w246) -> (w247:string[][])
          n105 = Transpose 2D Array(2D array=w247) -> (transposed array=w250:string[][])
          n106 = Number To Decimal String(number=w249) -> (decimal integer string=w251:string[])  [unwired: 1 in]
        }
      }
    }
    n107 = global read "VAR总磷氨氮全局变量.vi" "状态告警区"() -> (w86:T3)
    "总磷总氮运行状态" <- w86
    n108 = Unbundle By Name(w86) -> ("日志代码"=w73:u16)
    n109 = feedback-in #6(w73) -> ()
    n110 = feedback #6(w73) -> (w106:u16)
    n111 = Not Equal?(x=w73, y=w106) -> (x != y?=w105:bool)
    n112 = case shown="真" w105 {
      tunnel: w73 -> [_ w255]
      tunnel: w100 -> [_ w262]
      tunnel: w99 -> [_ w261]
      frame False {
      }
      frame True {
        n113 = Subtract(x=w255, y=1) -> (x-y=w253:i32)
        "多列列表框" <- w253
        n114 = Subtract(x=w253, y=5) -> (x-y=w257:i32)
        n115 = property on="多列列表框" class="MCListbox (严格)"("ItemNames"=w262, "RowHdrs[]"=w261) -> (error out=w263:errorcluster)  [unwired: 2 in, 1 out]
        n116 = Greater Or Equal To 0?(x=w257) -> (x >= 0?=w256:bool)
        n117 = property on="多列列表框" class="MCListbox (严格)"(error in=w263) -> (error out=w264:errorcluster, "TopLeft"=w265:T12)  [unwired: 1 in, 1 out]
        n118 = Select(t=w257, s=w256, f=0) -> (s? t:f=w258:i32)
        n119 = Bundle By Name(cluster=w265, "Row"=w258) -> (w266:T12)
        n120 = property on="多列列表框" class="MCListbox (严格)"(error in=w264, "TopLeft"=w266) -> ()  [unwired: 1 in, 2 out]
      }
    }
  }
  n121 = property class="VI"(reference=w32) -> ("Name"=w31:string)  [unwired: 1 in, 2 out]
  n122 = call "总磷氨氮MB_api.vi"("STEP"=enum16{"open", "read", "write", "close"}."open", "Error in"=w1) -> ("error out"=w8:errorcluster)  [unwired: 7 in, 2 out]
  n123 = Obtain Queue(name (unnamed)="NH3N" ("名称（未命名）"), element data type=cluster{"命令":string, "data":variant} {"命令"="", "data"=variant}) -> (queue out=w35:refnum<queue>, error out=w36:errorcluster)  [unwired: 3 in, 1 out]
  n124 = node-c288() -> (w6:T13)  [unwired: 4 in]
  n125 = property class="VI"(reference=w24) -> ("Name"=w17:string)  [unwired: 1 in, 2 out]
  n126 = control-ref of="测量模式下拉列表"() -> (w13:refnum<vi>)
  n127 = control-ref of="量程切换阈值"() -> (w11:refnum<vi>)
  n128 = control-ref of="参数下拉列表"() -> (w14:refnum<vi>)
  n129 = control-ref of="量程下拉列表"() -> (w15:refnum<vi>)
  n130 = timed-loop {
    timing: w6 -> [_]
    timing-out: [_] -> w5
    tunnel: w2 -> [w269]
    stop <- FALSE stop-if-true
    w270 = u16 3 items=["总磷"=1, "氨氮"=3] ("站号")
    # "定时更新"
    n131 = node-c288() -> ()  [unwired: 1 in, 1 out]
    n132 = call "总磷氨氮版本号读取.vi"() -> ("固件版本号"=→"固件版本号":string)  [unwired: 11 in]
    n133 = Bundle By Name(cluster=cluster{"命令":string, "data":variant} {"命令"="", "data"=variant} ("元素"), "命令"="读序列号", "data"=w270) -> (w268:cluster{"命令":string, "data":variant})
    n134 = Enqueue Element(queue=w269, element=w268) -> ()  [unwired: 2 in, 3 out]
    n135 = node-c288() -> ()  [unwired: 1 in, 1 out]
  }
  n136 = Open VI Reference(type specifier VI Refnum (for type only)=refnum<vi> refnum, vi path=w31, options=128 ("选项")) -> (vi reference=w29:refnum<vi>, error out=w27:errorcluster)  [unwired: 3 in]
  n137 = control-ref of="备用系数"() -> (w10:refnum<vi>)
  n138 = call-by-ref "?"(reference=w29, error in=w27) -> (reference out=w25:refnum<vi>, error out=w26:errorcluster)  [unwired: 12 in]
  n139 = control-ref of="公式"() -> (w12:refnum<vi>)
  n140 = Open VI Reference(type specifier VI Refnum (for type only)=refnum<vi> refnum, vi path=w17, options=128 ("选项")) -> (vi reference=w19:refnum<vi>, error out=w21:errorcluster)  [unwired: 3 in]
  n141 = Close Reference(reference=w25, error in (no error)=w26) -> ()  [unwired: 1 out]
  n142 = call-by-ref "?"(reference=w19, error in=w21) -> (reference out=w23:refnum<vi>, error out=w22:errorcluster)  [unwired: 12 in]
  n143 = while {
    tunnel: w35 -> [w278]
    shift-right: [w279] -> _
    shift-left: T4."待机" -> [w280]
    shift-right: [w276] -> _
    shift-left: u32 0 ("等待时间（毫秒）") -> [w277]
    stop <- FALSE stop-if-true
    n144 = Wait (ms)(milliseconds to wait=u32 1000 ("等待时间（毫秒）")) -> ()  [unwired: 1 out]
    n145 = local read "定时启动"() -> (w281:bool)
    n146 = case shown="真" w281 {
      tunnel: w280 -> [_ w289]
      tunnel: [T4."待机" w288] -> w279
      tunnel: w278 -> [_ w287]
      tunnel: w277 -> [_ w286]
      tunnel: [_ w285] -> w276
      frame False {
      }
      frame True {
        n147 = case shown="\"氨氮测量中\"" w289 {
          tunnel: [T4."启动氨氮" w294 w301 w312 w320 w332] -> w288
          tunnel: w287 -> [_ w299 _ w318 _ _]
          tunnel: w286 -> [_ _ _ _ _ w335]
          tunnel: [_ _ _ _ _ w331] -> w285
          frame "待机", Default {
          }
          frame "启动氨氮" {
            n148 = call "总磷氨氮启动命令.vi"("参数"=T16 {"站号"=3, "量程切换"=enum."AUTO", "控制命令"=enum."启动测量", "模式设置"=enum."待机", "测量间隔"=0}) -> ("启动命令"=w292:cluster{"命令":string, "data":variant})  [unwired: 10 in]
            n149 = Enqueue Element(queue=w299, element=w292) -> ()  [unwired: 2 in, 3 out]
            n150 = global read "VAR总磷氨氮全局变量.vi" "状态告警区"() -> (w298:T3)
            n151 = Unbundle By Name(w298) -> ("工作状态"=w297:T7)
            n152 = Not Equal To 0?(x=w297) -> (x != 0?=w296:bool)
            n153 = Select(t=T4."氨氮测量中", s=w296, f=T4."启动氨氮") -> (s? t:f=w294:T4)
          }
          frame "氨氮测量中" {
            n154 = flat-sequence {
              tunnel: [w305] -> w300
              tunnel: [w309] -> w301
              tunnel: w300 -> [w309]
              frame #0 {
                n155 = global read "VAR总磷氨氮全局变量.vi" "状态告警区"() -> (w306:T3)
                n156 = Unbundle By Name(w306) -> ("工作状态"=w307:T7)
                n157 = Equal To 0?(x=w307) -> (x = 0?=w302:bool)
                n158 = Select(t=T4."延时", s=w302, f=T4."氨氮测量中") -> (s? t:f=w305:T4)
              }
              frame #1 {
                n159 = Wait (ms)(milliseconds to wait=u32 5000 ("等待时间（毫秒）")) -> ()  [unwired: 1 out]
              }
            }
          }
          frame "启动总磷" {
            n160 = call "总磷氨氮启动命令.vi"("参数"=T16 {"站号"=1, "量程切换"=enum."AUTO", "控制命令"=enum."启动测量", "模式设置"=enum."待机", "测量间隔"=0}) -> ("启动命令"=w311:cluster{"命令":string, "data":variant})  [unwired: 10 in]
            n161 = Enqueue Element(queue=w318, element=w311) -> ()  [unwired: 2 in, 3 out]
            n162 = global read "VAR总磷氨氮全局变量.vi" "状态告警区"() -> (w313:T3)
            n163 = Unbundle By Name(w313) -> ("工作状态"=w314:T7)
            n164 = Not Equal To 0?(x=w314) -> (x != 0?=w315:bool)
            n165 = Select(t=T4."总磷测量中", s=w315, f=T4."启动总磷") -> (s? t:f=w312:T4)
          }
          frame "总磷测量中" {
            n166 = flat-sequence {
              tunnel: [w322] -> w319
              tunnel: [w328] -> w320
              tunnel: w319 -> [w328]
              frame #0 {
                n167 = global read "VAR总磷氨氮全局变量.vi" "状态告警区"() -> (w325:T3)
                n168 = Unbundle By Name(w325) -> ("工作状态"=w326:T7)
                n169 = Equal To 0?(x=w326) -> (x = 0?=w321:bool)
                n170 = Select(t=T4."延时", s=w321, f=T4."总磷测量中") -> (s? t:f=w322:T4)
              }
              frame #1 {
                n171 = Wait (ms)(milliseconds to wait=u32 5000 ("等待时间（毫秒）")) -> ()  [unwired: 1 out]
              }
            }
          }
          frame "延时" {
            n172 = local read "设置值"() -> (w334:dbl)
            n173 = Increment(x=w335) -> (x+1=w331:u32)
            n174 = Greater Or Equal?(x=w331, y=w334) -> (x >= y?=w333:bool)
            n175 = Select(t=T4."待机", s=w333, f=T4."延时") -> (s? t:f=w332:T4)
          }
        }
      }
    }
  }
  n176 = while {
    tunnel: w35 -> [w342]
    tunnel: w15 -> [w341]
    tunnel: w14 -> [w340]
    tunnel: w13 -> [w339]
    tunnel: w12 -> [w338]
    tunnel: w11 -> [w337]
    tunnel: w10 -> [w336]
    tunnel: w8 -> [_]
    stop <- FALSE stop-if-true
    n177 = event shown="[6] \"设置\": 值改变" {
      selector: _ -> [_ _ _ _ _ _ _ _ _ _ _ _ _ _ _ _]
      dyn-events: _ -> [_ _ _ _ _ _ _ _ _ _ _ _ _ _ _ _]
      timeout: _ -> [_ _ _ _ _ _ _ _ _ _ _ _ _ _ _ _]
      tunnel: w342 -> [_ w346 _ w357 w359 _ _ _ _ _ _ _ _ _ _ _]
      tunnel: w341 -> [_ _ _ _ _ _ _ _ _ _ w413 _ w433 w442 _ _]
      tunnel: w340 -> [_ _ _ _ _ _ _ _ _ _ w411 _ w431 w444 w452 w459]
      tunnel: w339 -> [_ _ _ _ _ _ _ _ _ _ w412 _ w432 w443 _ _]
      tunnel: w338 -> [_ _ _ _ _ _ _ _ _ _ w407 _ _ _ _ _]
      tunnel: w337 -> [_ _ _ _ _ _ _ _ _ _ _ _ w427 _ _ _]
      tunnel: w336 -> [_ _ _ _ _ _ _ _ _ _ _ _ _ _ w450 _]
      event Timeout {
        n178 = event-data() -> ()  [unwired: 1 in, 3 out]
      }
      event "手动启动": Value Change {
        n179 = event-data() -> ()  [unwired: 1 in, 6 out]
        n180 = call "总磷氨氮启动参数对话框.vi"() -> ("确认"=w344:bool, "元素"=w345:cluster{"命令":string, "data":variant})  [unwired: 10 in]
        n181 = case shown="真" w344 {
          tunnel: w346 -> [_ w348]
          tunnel: w345 -> [_ w347]
          frame False {
          }
          frame True {
            n182 = Enqueue Element(queue=w348, element=w347) -> ()  [unwired: 2 in, 3 out]
          }
        }
      }
      event "定时启动": Mouse Down {
        n183 = event-data() -> ()  [unwired: 1 in, 6 out]
        n184 = call "定时启动对话框.vi"() -> ("设置值"=→"设置值":dbl, "确定输出"=→"定时启动":bool)  [unwired: 10 in]
      }
      event "单步测试": Value Change {
        w352 = u16 1 items=["总磷"=1, "氨氮"=3] ("站号")
        n185 = event-data() -> ()  [unwired: 1 in, 6 out]
        n186 = Bundle("站号"=w352, "总磷氨氮调试"="总磷氨氮调试") -> (w351:cluster{"站号":u16, "总磷氨氮调试":u16[]})  [unwired: 1 in]
        n187 = Bundle By Name(cluster=cluster{"命令":string, "data":variant} {"命令"="", "data"=variant} ("元素"), "命令"="debug", "data"=w351) -> (w354:cluster{"命令":string, "data":variant})
        n188 = Enqueue Element(queue=w357, element=w354) -> ()  [unwired: 2 in, 3 out]
      }
      event "停止": Value Change {
        n189 = event-data() -> ()  [unwired: 1 in, 6 out]
        n190 = Enqueue Element(queue=w359, element=cluster{"命令":string, "data":variant} {"命令"="启动", "data"=variant(cluster{"站号":u16, "控制命令输出":u16[]} {"站号"=1, "控制命令输出"=[2816]})} ("元素")) -> ()  [unwired: 2 in, 3 out]
      }
      event "调试": Value Change {
        n191 = event-data() -> ()  [unwired: 1 in, 6 out]
        n192 = property on="窗格" class="Pane"("Origin"=T5 {"Horizontal"=0, "Vertical"=528} ("原点")) -> ()  [unwired: 2 in, 2 out]
      }
      event "设置": Value Change {
        n193 = event-data() -> ()  [unwired: 1 in, 6 out]
        n194 = property on="窗格" class="Pane"("Origin"=T5 {"Horizontal"=0, "Vertical"=1256} ("原点")) -> ()  [unwired: 2 in, 2 out]
      }
      event "返回", "返回 2": Value Change {
        n195 = event-data() -> ()  [unwired: 1 in, 6 out]
        n196 = property on="窗格" class="Pane"("Origin"=T5 {"Horizontal"=0, "Vertical"=0} ("原点")) -> ()  [unwired: 2 in, 2 out]
      }
      event "标液浓度1", "测量吸光度1", "测量吸光度2", "标液浓度2", "测量吸光度3", "标液浓度3", "测量吸光度4", "标液浓度4", "测量吸光度5", "标液浓度5", "样品1启用", "样品3启用", "样品4启用", "样品5启用", "样品2启用", "模型", "method", "样品1 F0", "样品1 F1", "样品2 F1", "样品2 F0", "样品3 F1", "样品4 F0", "样品4 F1", "样品5 F1", "样品5 F0", "精度": Value Change {
        n197 = event-data() -> ()  [unwired: 1 in, 6 out]
        n198 = formula code="E=log(F0/F1);"("F0"="样品1 F0", "F1"="样品1 F1") -> ("E"=w384:dbl)
        "测量吸光度1" <- w384
        n199 = formula code="E=log(F0/F1);"("F0"="样品2 F0", "F1"="样品2 F1") -> ("E"=w381:dbl)
        "测量吸光度2" <- w381
        n200 = formula code="E=log(F0/F1);"("F0"="样品3 F0", "F1"="样品3 F1") -> ("E"=w378:dbl)
        "测量吸光度3" <- w378
        n201 = formula code="E=log(F0/F1);"("F0"="样品4 F0", "F1"="样品4 F1") -> ("E"=w375:dbl)
        "测量吸光度4" <- w375
        n202 = formula code="E=log(F0/F1);"("F0"="样品5 F0", "F1"="样品5 F1") -> ("E"=w372:dbl)
        "测量吸光度5" <- w372
        n203 = Replace Array Subset(array=dbl[] [0.0, 0.0, 0.0, 0.0, 0.0] ("数组"), new element #1="标液浓度1", new element #2="标液浓度2", new element #3="标液浓度3", new element #4="标液浓度4", new element #5="标液浓度5") -> (w369:dbl[])  [unwired: 5 in]
        n204 = Replace Array Subset(array=dbl[] [0.0, 0.0, 0.0, 0.0, 0.0] ("数组"), new element #1=w384, new element #2=w381, new element #3=w378, new element #4=w375, new element #5=w372) -> (w368:dbl[])  [unwired: 5 in]
        n205 = Replace Array Subset(array=bool[] [FALSE, FALSE, FALSE, FALSE, FALSE] ("数组"), new element #1="样品1启用", new element #2="样品2启用", new element #3="样品3启用", new element #4="样品4启用", new element #5="样品5启用") -> (w367:bool[])  [unwired: 5 in]
        n206 = call "线性公式.vi"("精度"="精度", "模型"="模型", "method"="method", "启用"=w367, "监测浓度"=w368, "标液浓度"=w369) -> ("XY图"=→"XY图":cluster{"X Values":dbl[], "Y Values":dbl[]}[], "r^2"=→"r^2":dbl, "拟合方程"=→"拟合公式":string)  [unwired: 3 in]
      }
      event "标液浓度1", "标液浓度2", "标液浓度3", "标液浓度4", "标液浓度5", "样品1 F0", "样品1 F1", "样品2 F1", "样品2 F0", "样品3 F1", "样品3 F0", "样品4 F0", "样品4 F1", "样品5 F0", "样品5 F1", "精度", "公式.X^2", "公式.X", "公式.b", "量程切换阈值.阈值", "量程切换阈值.标液浓度", "备用系数.量程上限", "备用系数.量程下限", "备用系数.检出限", "备用系数.精度": Mouse Down {
        n207 = event-data() -> ("CtlRef"=w403:refnum<vi>)  [unwired: 1 in, 5 out]
        n208 = property class="DigNum (严格)"(reference=w403) -> (reference out=w401:refnum<vi>, "Value"=w402:dbl)  [unwired: 1 in, 1 out]
        n209 = call "数字键盘.vi"("OldNumber"=w402) -> ("NewNumber"=w400:sgl)
        n210 = property class="DigNum (严格)"(reference=w401, "Val(Sgnl)"=w400) -> ()  [unwired: 1 in, 2 out]
      }
      event "读公式": Value Change {
        n211 = event-data() -> ()  [unwired: 1 in, 6 out]
        n212 = property class="Enum (严格)"(reference=w411) -> ("Value"=w410:enum16{"氨氮", "总磷"})  [unwired: 1 in, 2 out]
        n213 = property class="Enum (严格)"(reference=w412) -> ("Value"=w409:enum16{"水样测量", "空白核查", "标样核查", "盲样测试", "加标回收"})  [unwired: 1 in, 2 out]
        n214 = property class="Enum (严格)"(reference=w413) -> ("Value"=w408:enum16{"低量程", "高量程"})  [unwired: 1 in, 2 out]
        n215 = call "总磷氨氮公式读取.vi"("量程"=w408, "测量模式"=w409, "测量参数"=w410) -> ("error out"=w405:errorcluster, "公式"=w406:cluster{"X^2":dbl, "X":dbl, "b":dbl})  [unwired: 7 in]
        n216 = property class="Clust (严格)"(reference=w407, "Value"=w406) -> ()  [unwired: 1 in, 2 out]
        n217 = case shown="错误" w405 {
          tunnel: ["读取成功" ("消息") "读取失败" ("消息")] -> w404
          frame No Error {
          }
          frame Error {
          }
        }
        n218 = One Button Dialog(message=w404) -> ()  [unwired: 1 in, 1 out]
      }
      event "写公式": Value Change {
        n219 = event-data() -> ()  [unwired: 1 in, 6 out]
        n220 = call "总磷氨氮公式写入.vi"("公式"="公式", "量程"="量程下拉列表", "测量模式"="测量模式下拉列表", "测量参数"="参数下拉列表") -> ("error out"=w416:errorcluster)  [unwired: 7 in]
        n221 = case shown="无错误" w416 {
          tunnel: ["写入成功" ("消息") "写入失败" ("消息")] -> w417
          frame No Error {
          }
          frame Error {
          }
        }
        n222 = One Button Dialog(message=w417) -> ()  [unwired: 1 in, 1 out]
      }
      event "量程切换阈值读取": Value Change {
        n223 = event-data() -> ()  [unwired: 1 in, 6 out]
        n224 = property class="Enum (严格)"(reference=w431) -> ("Value"=w430:enum16{"氨氮", "总磷"})  [unwired: 1 in, 2 out]
        n225 = property class="Enum (严格)"(reference=w432) -> ("Value"=w429:enum16{"水样测量", "空白核查", "标样核查", "盲样测试", "加标回收"})  [unwired: 1 in, 2 out]
        n226 = property class="Enum (严格)"(reference=w433) -> ("Value"=w428:enum16{"低量程", "高量程"})  [unwired: 1 in, 2 out]
        n227 = call "总磷氨氮量程读取.vi"("量程"=w428, "测量模式"=w429, "测量参数"=w430) -> ("error out"=w424:errorcluster, "量程切换阈值"=w426:cluster{"阈值":dbl, "标液浓度":dbl})  [unwired: 7 in]
        n228 = property class="Clust (严格)"(reference=w427, "Value"=w426) -> ()  [unwired: 1 in, 2 out]
        n229 = case shown="错误" w424 {
          tunnel: ["读取成功" ("消息") "读取失败" ("消息")] -> w425
          frame No Error {
          }
          frame Error {
          }
        }
        n230 = One Button Dialog(message=w425) -> ()  [unwired: 1 in, 1 out]
      }
      event "量程切换阈值写入": Value Change {
        n231 = event-data() -> ()  [unwired: 1 in, 6 out]
        n232 = property class="Enum (严格)"(reference=w444) -> ("Value"=w441:enum16{"氨氮", "总磷"})  [unwired: 1 in, 2 out]
        n233 = property class="Enum (严格)"(reference=w443) -> ("Value"=w440:enum16{"水样测量", "空白核查", "标样核查", "盲样测试", "加标回收"})  [unwired: 1 in, 2 out]
        n234 = property class="Enum (严格)"(reference=w442) -> ("Value"=w439:enum16{"低量程", "高量程"})  [unwired: 1 in, 2 out]
        n235 = call "总磷氨氮量程写入.vi"("量程切换阈值"="量程切换阈值", "量程"=w439, "测量模式"=w440, "测量参数"=w441) -> ("error out"=w436:errorcluster)  [unwired: 7 in]
        n236 = case shown="无错误" w436 {
          tunnel: ["写入成功" ("消息") "写入失败" ("消息")] -> w437
          frame No Error {
          }
          frame Error {
          }
        }
        n237 = One Button Dialog(message=w437) -> ()  [unwired: 1 in, 1 out]
      }
      event "备用系数读取": Value Change {
        n238 = event-data() -> ()  [unwired: 1 in, 6 out]
        n239 = property class="Enum (严格)"(reference=w452) -> ("Value"=w451:enum16{"氨氮", "总磷"})  [unwired: 1 in, 2 out]
        n240 = call "总磷氨氮备用系数读取.vi"("测量参数"=w451) -> ("error out"=w447:errorcluster, "备用系数"=w449:T1)  [unwired: 9 in]
        n241 = property class="Clust (严格)"(reference=w450, "Value"=w449) -> ()  [unwired: 1 in, 2 out]
        n242 = case shown="错误" w447 {
          tunnel: ["读取成功" ("消息") "读取失败" ("消息")] -> w448
          frame No Error {
          }
          frame Error {
          }
        }
        n243 = One Button Dialog(message=w448) -> ()  [unwired: 1 in, 1 out]
      }
      event "备用系数写入": Value Change {
        n244 = event-data() -> ()  [unwired: 1 in, 6 out]
        n245 = property class="Enum (严格)"(reference=w459) -> ("Value"=w458:enum16{"氨氮", "总磷"})  [unwired: 1 in, 2 out]
        n246 = call "总磷氨氮备用系数写入.vi"("备用系数"="备用系数", "测量参数"=w458) -> ("error out"=w455:errorcluster)  [unwired: 9 in]
        n247 = case shown="无错误" w455 {
          tunnel: ["写入成功" ("消息") "写入失败" ("消息")] -> w456
          frame No Error {
          }
          frame Error {
          }
        }
        n248 = One Button Dialog(message=w456) -> ()  [unwired: 1 in, 1 out]
      }
    }
  }
  n249 = while {
    tunnel: w35 -> [w477]
    tunnel: w36 -> [_]
    shift-right: [w471] -> _
    shift-left: enum16{"氨氮", "总磷"}."氨氮" ("枚举") -> [w472]
    stop <- FALSE stop-if-true
    w470 = u16 3 items=["总磷"=1, "氨氮"=3] ("站号")
    # "试剂填充 172 \n管路清洗108\n氨氮92\n总磷131\n总磷海水147\n总氮76\n总氮海水92"
    n250 = Wait (ms)(milliseconds to wait=u32 1000 ("等待时间（毫秒）")) -> ()  [unwired: 1 out]
    n251 = global read "VAR总磷氨氮全局变量.vi" "状态告警区"() -> (w468:T3)
    n252 = Bundle By Name(cluster=cluster{"命令":string, "data":variant} {"命令"="", "data"=variant} ("元素"), "命令"="读状态告警区", "data"=w470) -> (w479:cluster{"命令":string, "data":variant})
    n253 = Unbundle By Name(w468) -> ("系统时间"=w467:timestamp)
    n254 = Bundle By Name(cluster=cluster{"命令":string, "data":variant} {"命令"="", "data"=variant} ("元素"), "命令"="读测量数据区", "data"=w470) -> (w475:cluster{"命令":string, "data":variant})
    n255 = Enqueue Element(queue=w477, element=w479) -> (queue out=w473:refnum<queue>)  [unwired: 2 in, 2 out]
    n256 = Get Date/Time In Seconds() -> (seconds since 1Jan1904=w466:timestamp)
    n257 = Subtract(x=w466, y=w467) -> (x-y=w465:dbl)
    n258 = Enqueue Element(queue=w473, element=w475) -> (queue out=w469:refnum<queue>)  [unwired: 2 in, 2 out]
    n259 = Absolute Value(x=w465) -> (abs(x)=w464:dbl)
    n260 = Greater Or Equal?(x=w464, y=120.0) -> (x >= y?=w462:bool)
    n261 = case shown="真" w462 {
      tunnel: w469 -> [_ w484]
      frame False {
      }
      frame True {
        n262 = call "总磷氨氮启动命令.vi"("参数"=T17 {"站号"=3, "量程切换"=enum."AUTO", "控制命令"=enum."校时", "模式设置"=enum."待机", "测量间隔"=0}) -> ("启动命令"=w483:cluster{"命令":string, "data":variant})  [unwired: 10 in]
        n263 = Enqueue Element(queue=w484, element=w483) -> ()  [unwired: 2 in, 3 out]
      }
    }
    n264 = Increment(x=w472) -> (x+1=w471:enum16{"氨氮", "总磷"})
  }
  n265 = Close Reference(reference=w23, error in (no error)=w22) -> ()  [unwired: 1 out]
  n266 = node-c288(w5) -> ()  [unwired: 1 out]
